vi "save sample data.vi"(0 "Sample cluster":T1={"General description"="", "Sample setup"={"integration time"=0.5, "rinse time"=10.0, "sample time"=10.0, "sample type"=0}, "Absorbance"=[], "Analyst"="", "Sample descriptions"=[], "good data"=[]} {"Absorbance" format="%.2e"; "Sample setup"."sample type" items=["Sample Cuvet", "Sipper Cell", "No Dialog"]; "Sample setup"."sample time" min=0.0 max=100.0 step=1.0 format="%.1f"; "Sample setup"."rinse time" min=0.0 max=100.0 step=1.0 format="%.1f"; "Sample setup"."integration time" format="%.1f"}) -> ()   [LabVIEW 2015]
uses:
  sample cluster.ctl
  settings.ctl
  file/file action.ctl
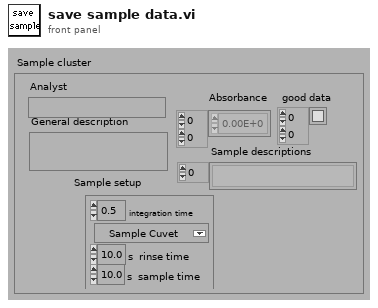
[diagram p1: front panel]
types:
  T1 = typedef "sample cluster.ctl" = cluster{"General description":string, "Sample setup":T2, "Absorbance":dbl[][], "Analyst":string, "Sample descriptions":string[], "good data":bool[][]}
  T2 = typedef "settings.ctl" = cluster{"integration time":sgl, "rinse time":dbl[unit], "sample time":dbl[unit], "sample type":u16}
  T3 = typedef "file action.ctl" = enum16{"Save", "Open"}
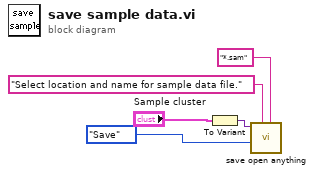
[diagram p0: block diagram]
diagram:
  n1 = To Variant(anything="Sample cluster") -> (Variant=w3:variant)
  n2 = call "save open anything.vi"("Variant"=w3, "Action"=file_action."Save", "prompt"="Select location and name for sample data file.", "pattern"="*.sam") -> ()  [unwired: 3 in, 4 out]
